vi "LVFunction_Imop_HIMG file_GetInformation.vi"(0 "Configuration file path":path, 11 "error in (no error)":errorcluster) -> (4 "Configuration file path (dup)":path, 6 "Image info":T1={"HasoSerialNumber"="", "CameraNumber"="", "Number of bits"=enum."16", "Size"={"X"=0, "Y"=0}, "Time Stamp"=timestamp(0 s since 1904-01-01), "Number of summed images"=0, "Exposure duration spe (us)"=0, "Exposure duration real (us)"=0, "Gain"=0.0}, 15 "error out":errorcluster)   [LabVIEW 2020]
doc: "Get acquisition information from image file.\n\n--------------------------------------------------------------------------------\n\n<B>image_file_pathIn</B> : Absolute path to image file.\n<B>image_file_pathOut</B> : Absolute path to image file.\n<B>bit_depth</B> : Image bits depth.\n<B>size</B> : Image size.\n<B>time_stamp</B> : Acquisition time.\n<B>haso_serial_number</B> : Haso serial number.\n<B>camera_serial_number</B> : Camera serial number.\n<B>em_ccd_gain</B> : Emccd gain.\n<B>nb_summed_images</B> : Number summed image.\n<B>exposure_time_requested</B> : Exposure duration requested (us).\n<B>exposure_time_applied</B> : Exposure duration applied (us).\n<B>ErrorIn</B> : Error\n<B>ErrorOut</B> : Error\n\n--------------------------------------------------------------------------------"
uses:
  Controls/HIMG File information.ctl
  Controls/Data alignment enum.ctl
  Controls/Point2D.ctl
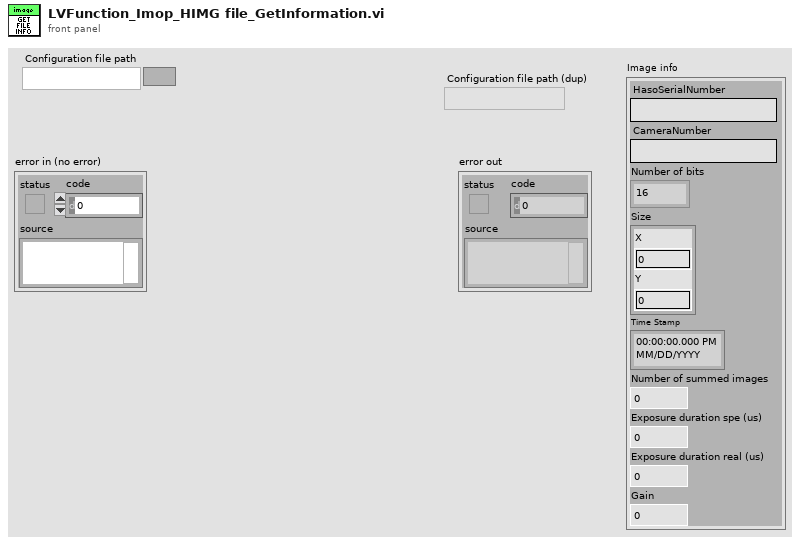
[diagram p1: front panel]
types:
  T1 = typedef "HIMG File information.ctl" = cluster{"HasoSerialNumber":string, "CameraNumber":string, "Number of bits":T2, "Size":T3, "Time Stamp":timestamp, "Number of summed images":i32, "Exposure duration spe (us)":i32, "Exposure duration real (us)":i32, "Gain":sgl}
  T2 = typedef "Data alignment enum.ctl" = enum16{"8", "16", "32"}
  T3 = typedef "Point2D.ctl" = cluster{"X":u32, "Y":u32}
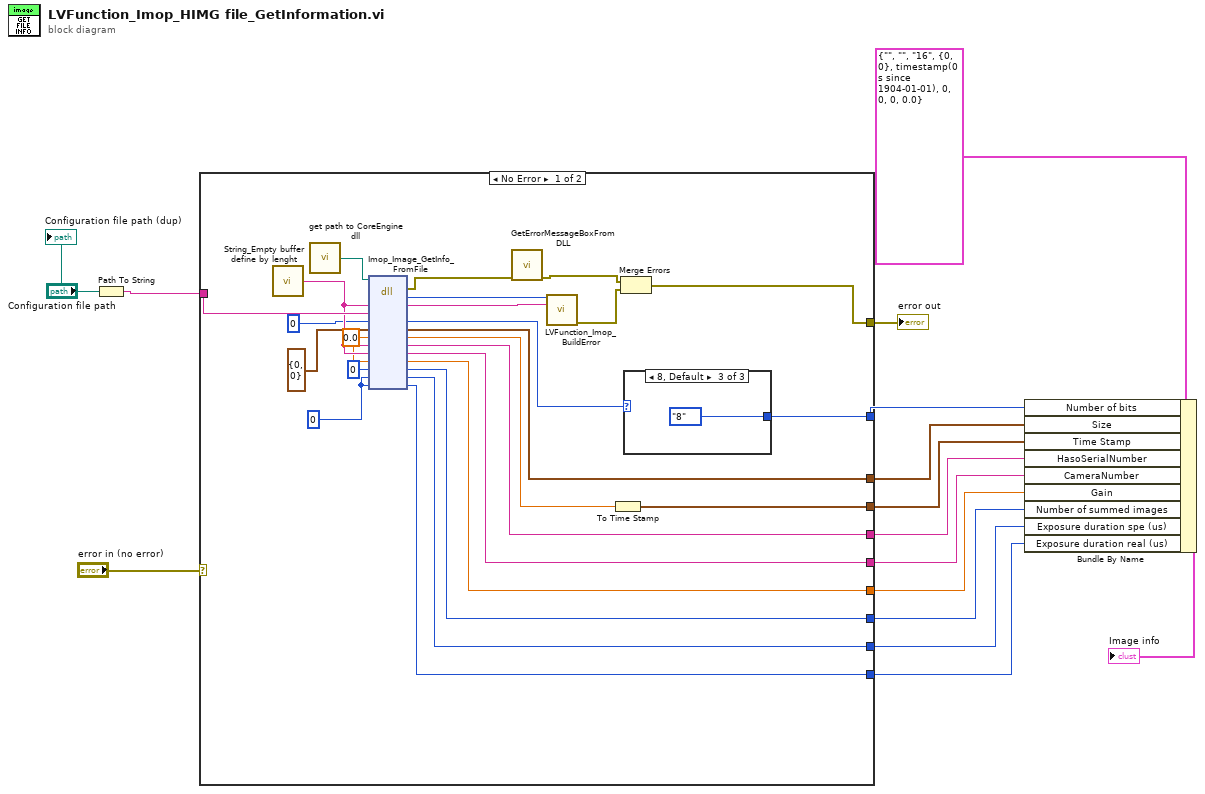
[diagram p0: block diagram]
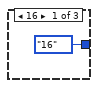
[diagram p2: hidden frame]
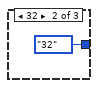
[diagram p3: hidden frame]
diagram:
  n1 = Path To String(path="Configuration file path") -> (string=w13:string)
  n2 = case shown="No Error" "error in (no error)" {
    selector: "error in (no error)" -> [_ w44]
    tunnel: [w23 w44] -> w14
    tunnel: [w36 _] -> w8
    tunnel: w13 -> [w34 _]
    tunnel: [w32 _] -> w5
    tunnel: [w30 _] -> w9
    tunnel: [w29 _] -> w6
    tunnel: [w26 _] -> w7
    tunnel: [w20 _] -> w4
    tunnel: [w19 _] -> w3
    tunnel: [w17 _] -> w2
    tunnel: [w16 _] -> w1
    frame No Error {
      w18 = 0 ("Exposure duartion_spe_micros")
      w22 = 0.0 ("TimeStamp")
      n3 = call "String_Empty buffer define by lenght.vi"() -> ("Empty buffer"=w33:string)  [unwired: 1 in]
      n4 = call "get path to CoreEngine dll.vi"() -> ("path to wavekit library"=w38:path)  [unwired: 14 in, 1 out]
      n5 = dll-call lib="D:/2_trunk/temp_core_engine/DLLs/ImopEngine4_vc100.dll" fn="Imop_Image_GetInfo_FromFile"(path in=w38, "message"=w33, "path"=w34, "type"=u16 0, "size"=T3 {"X"=0, "Y"=0} ("Size"), "TimeStamp"=w22, "HasoSerialNumber"=w33, "CameraNumber"=w33, "gain"=w22, "Nbimage"=u32 0, "Exposure duartion_spe_micros"=w18, "Exposure duartion_micros"=w18) -> (error out=w37:errorcluster, "return type"=w40:i32, "message"=w39:string, "type"=w31:u16, "size"=w36:T3, "TimeStamp"=w27:dbl, "HasoSerialNumber"=w32:string, "CameraNumber"=w29:string, "gain"=w20:sgl, "Nbimage"=w19:u32, "Exposure duartion_spe_micros"=w17:u32, "Exposure duartion_micros"=w16:u32)  [unwired: 3 in, 1 out]
      n6 = call "GetErrorMessageBoxFromDLL.vi"("error IN"=w37) -> ("error OUT"=w25:errorcluster)  [unwired: 10 in]
      n7 = call "LVFunction_Imop_BuildError.vi"("code"=w40, "String to Prepend to source (\"\")"=w39) -> ("error out"=w24:errorcluster)  [unwired: 13 in]
      n8 = To Time Stamp(1:w27) -> (0:w26:timestamp)
      n9 = Merge Errors(w25, w24) -> (w23:errorcluster)
      n10 = case shown="8, Default" w31 {
        tunnel: [Data_alignment_enum."16" ("Number of bits") Data_alignment_enum."32" ("Number of bits") Data_alignment_enum."8" ("Number of bits")] -> w30
        frame 16 {
        }
        frame 32 {
        }
        frame 8, Default {
        }
      }
    }
    frame Error {
    }
  }
  "error out" <- w14
  n11 = Bundle By Name(cluster=T1 {"HasoSerialNumber"="", "CameraNumber"="", "Number of bits"=enum."16", "Size"={"X"=0, "Y"=0}, "Time Stamp"=timestamp(0 s since 1904-01-01), "Number of summed images"=0, "Exposure duration spe (us)"=0, "Exposure duration real (us)"=0, "Gain"=0.0} ("Cluster"), "Number of bits"=w9, "Size"=w8, "Time Stamp"=w7, "HasoSerialNumber"=w5, "CameraNumber"=w6, "Gain"=w4, "Number of summed images"=w3, "Exposure duration spe (us)"=w2, "Exposure duration real (us)"=w1) -> (→"Image info":T1)
  "Configuration file path (dup)" <- "Configuration file path"
